vi "Calculate Zoom Factor.vi"(9 "image data":T1, 10 "Draw Area Size":T2) -> (2 "Zoom Factor":dbl)   [LabVIEW 2020]
uses:
  <vilib>/Utility/miscctls.llb/LVBoundsTypeDef.ctl
  <vilib>/picture/picture.llb/imagedata.ctl
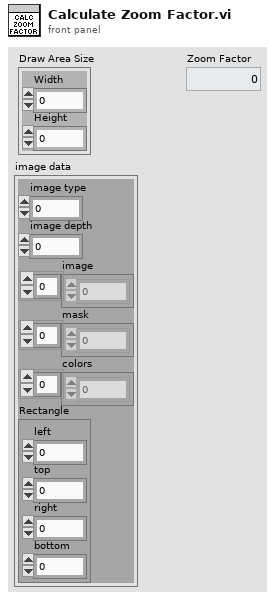
[diagram p1: front panel]
types:
  T1 = typedef "imagedata.ctl" = cluster{"image type":i32, "image depth":i32, "image":u8[], "mask":u8[], "colors":u32[], "Rectangle":cluster{"left":i16, "top":i16, "right":i16, "bottom":i16}}
  T2 = typedef "LVBoundsTypeDef.ctl" = cluster{"Width":u32, "Height":u32}
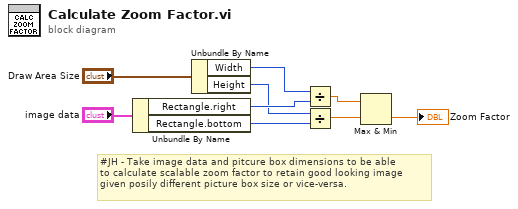
[diagram p0: block diagram]
diagram:
  # "#JH - Take image data and pitcure box dimensions to be able\nto calculate scalable zoom factor to retain good looking image\ngiven posily different picture box size or vice-versa."
  n1 = Unbundle By Name("image data") -> ("Rectangle.right"=w4:i16, "Rectangle.bottom"=w3:i16)
  n2 = Unbundle By Name("Draw Area Size") -> ("Width"=w1:u32, "Height"=w2:u32)
  n3 = Divide(x=w1, y=w4) -> (x/y=w5:dbl)
  n4 = Divide(x=w2, y=w3) -> (x/y=w6:dbl)
  n5 = Max & Min(x=w5, y=w6) -> (min(x,y)=→"Zoom Factor":dbl)  [unwired: 1 out]
